vi "IR_Wavelength_Tuning.vi"(7 "Wavelength (nm)":dbl) -> (15 "error_Code":i32)   [LabVIEW 2015]
uses:
  OPOTEK.dll
panel:
  # "WAVELENGTH TUNING"
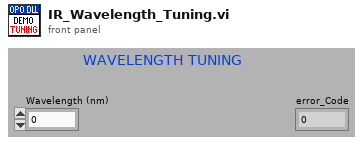
[diagram p1: front panel]
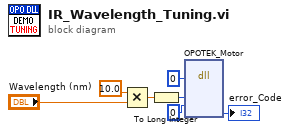
[diagram p0: block diagram]
diagram:
  n1 = Multiply(x=10.0, y="Wavelength (nm)") -> (x*y=w4:dbl)
  n2 = To Long Integer(number=w4) -> (32bit integer=w5:i32)
  n3 = dll-call lib="Z:/Software/Labview/FD_VIs/IR Opolette Controller/OPOTEK.dll" fn="OPOTEK_Motor"("action"=i8 0, "parameter1"=w5, "parameter2"=0) -> ("error_Code"=→"error_Code":i32)  [unwired: 8 in, 2 out]
